vi "FFT done for one mic.vi"() -> ()   [LabVIEW 2021]
uses:
  <vilib>/Analysis/2dsp.llb/Real FFT.vi
  <vilib>/express/express analysis/Spectral/Block/exnSpectralBlock spectral measurements RMS poly.vi
  <vilib>/express/express analysis/Spectral/Block/exnSpectralBlock spectral measurements RMS DDT.vi
  <vilib>/express/express analysis/Spectral/XNode/ExpressSpectralMeasurementsBlockNode.xnode
  <vilib>/Analysis/NI_AALPro.lvlib
panel:
  out "Waveform Graph":dbl[][](graph)
  out "Waveform Chart 3":dynamicdata(graph)
  out "Waveform Chart 2":dbl[](graph)
  out "Waveform Chart":dynamicdata(graph)
  in  "FFT size":i32=-1
  out "Numeric":dbl
  in  "stop (F)":bool
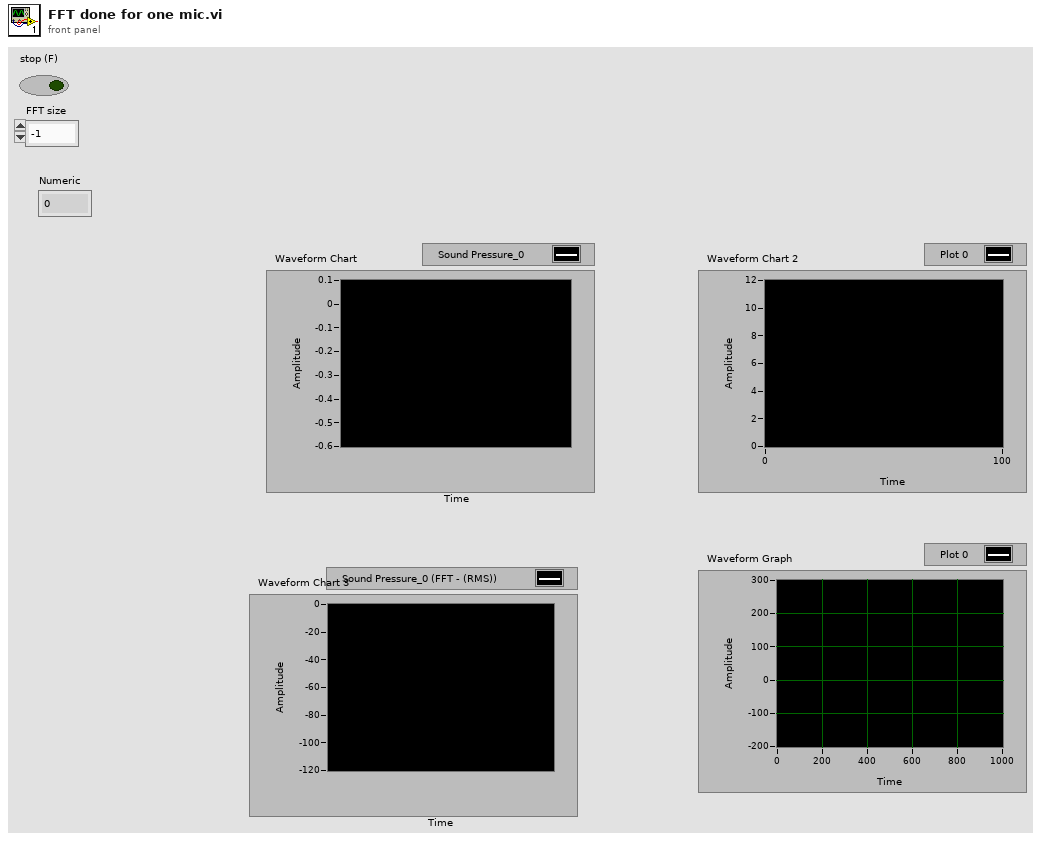
[diagram p1: front panel]
types:
  T1 = cluster{"averaging mode":u16, "weighting mode":u16, "number of averages":u32}
  T2 = cluster{"dB On (F)":bool, "unwrap phase (F)":bool, "convert to degree (F)":bool}
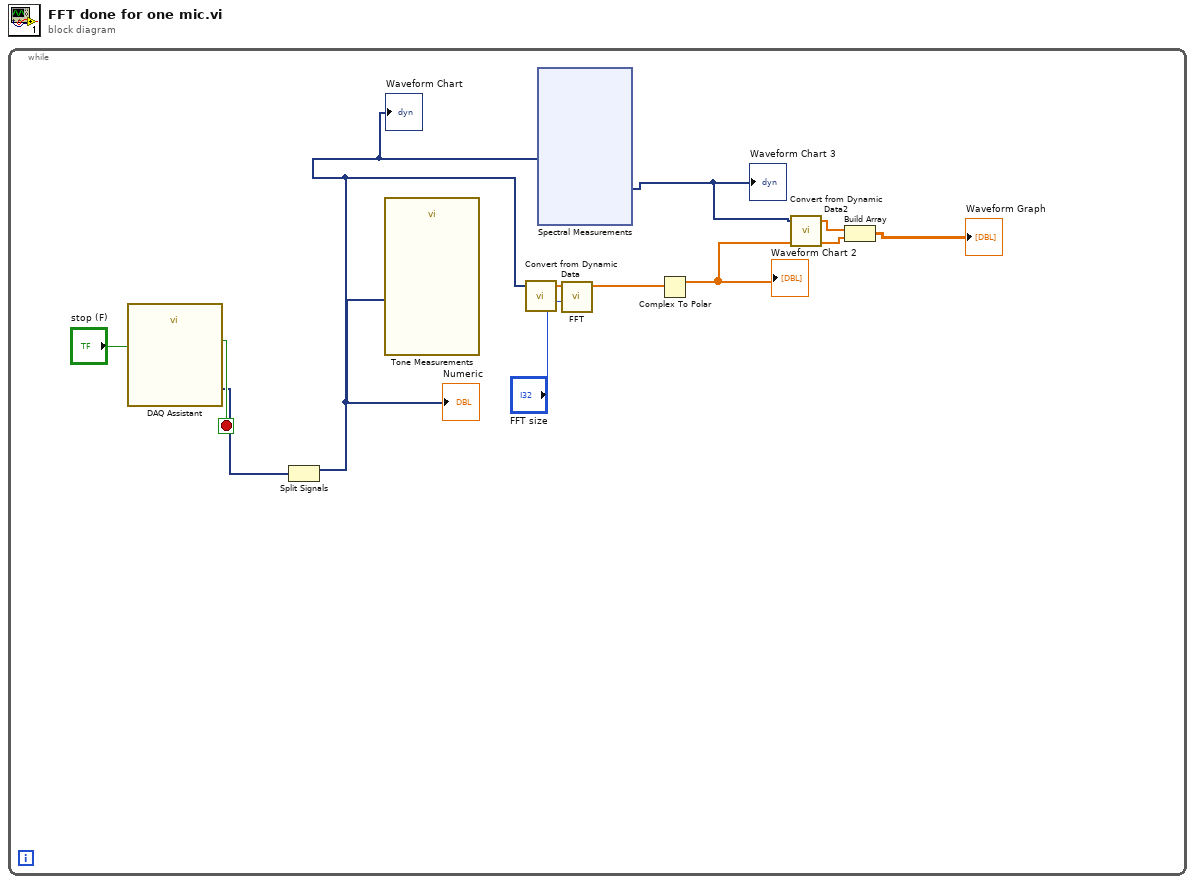
[diagram p0: block diagram]
diagram:
  n1 = while {
    stop <- w10 stop-if-true
    n2 = call "DAQ Assistant"("stop (F)"="stop (F)") -> ("data"=w9:dynamicdata, "stopped"=w10:bool)  [unwired: 15 in, 2 out]
    n3 = Split Signals(w9) -> (w6:dynamicdata)  [unwired: 2 in, 1 out]
    "Numeric" <- w6
    "Waveform Chart" <- w6
    n4 = call "Tone Measurements"("Signals"=w6) -> ()  [unwired: 8 in, 3 out]
    n5 = call "Convert from Dynamic Data"("Dynamic Data Type"=w6) -> ("Array"=w7:dbl[])  [unwired: 3 in]
    n6 = xnode "Spectral Measurements"("Signals"=w6) -> ("FFT - (RMS)"=w3:dynamicdata)  [unwired: 1 in, 2 out]
    "Waveform Chart 3" <- w3
    n7 = call-poly <vilib>:"FFT.vi"("FFT size"="FFT size", "X"=w7) -> ("FFT {X}"=w5:cdb[])  [unwired: 8 in, 1 out]
    n8 = Complex To Polar(r * e^(i*theta)=w5) -> (r=w4:dbl[])  [unwired: 1 out]
    "Waveform Chart 2" <- w4
    n9 = call "Convert from Dynamic Data2"("Dynamic Data Type"=w3) -> ("Array"=w2:dbl[])  [unwired: 3 in]
    n10 = Build Array(w2, w4) -> (→"Waveform Graph":dbl[][])
  }
